vi "Image Processing.vi"(0 "File Path":path=path "C:/General AFM lithography program/Sample.ibw", 1 "Lithography Information":T2(array[cluster])=array7x3944[27608 elements], 2 "Crop?":bool, 3 "Crop Data":T3, 4 "Angle (degrees)":dbl, 5 "error in (no error)":errorcluster, 6 "Size":cluster{"Width":dbl, "Height":dbl}={"Width"=40.0, "Height"=40.0}, 7 "Page":i32=1, 11 "Resolution":i32=1024) -> (14 "Image Out":T4(plugin-control), 15 "Offset":T1={"X Offset (µm)"=-1.2812, "Y Offset (µm)"=5.2969}, 16 "Sample Size":cluster{"Width (µm)":dbl, "Height (µm)":dbl}={"Width (µm)"=40.0, "Height (µm)"=40.0}, 19 "error out":errorcluster)   [LabVIEW 2013]
uses:
  <vilib>/vision/NI_Vision_Development_Module.lvlib
panel:
  out "Suggested max":dbl
  out "Suggested min":dbl
  in  "Interested image data max":dbl(slide) min=-6.03287162448396e-08 max=6.376236569849425e-07 scale=-6.03287162448396e-08..6.376236569849425e-07
  in  "Interested image data min":dbl(slide) min=-6.03287162448396e-08 max=6.376236569849425e-07 scale=-6.03287162448396e-08..6.376236569849425e-07
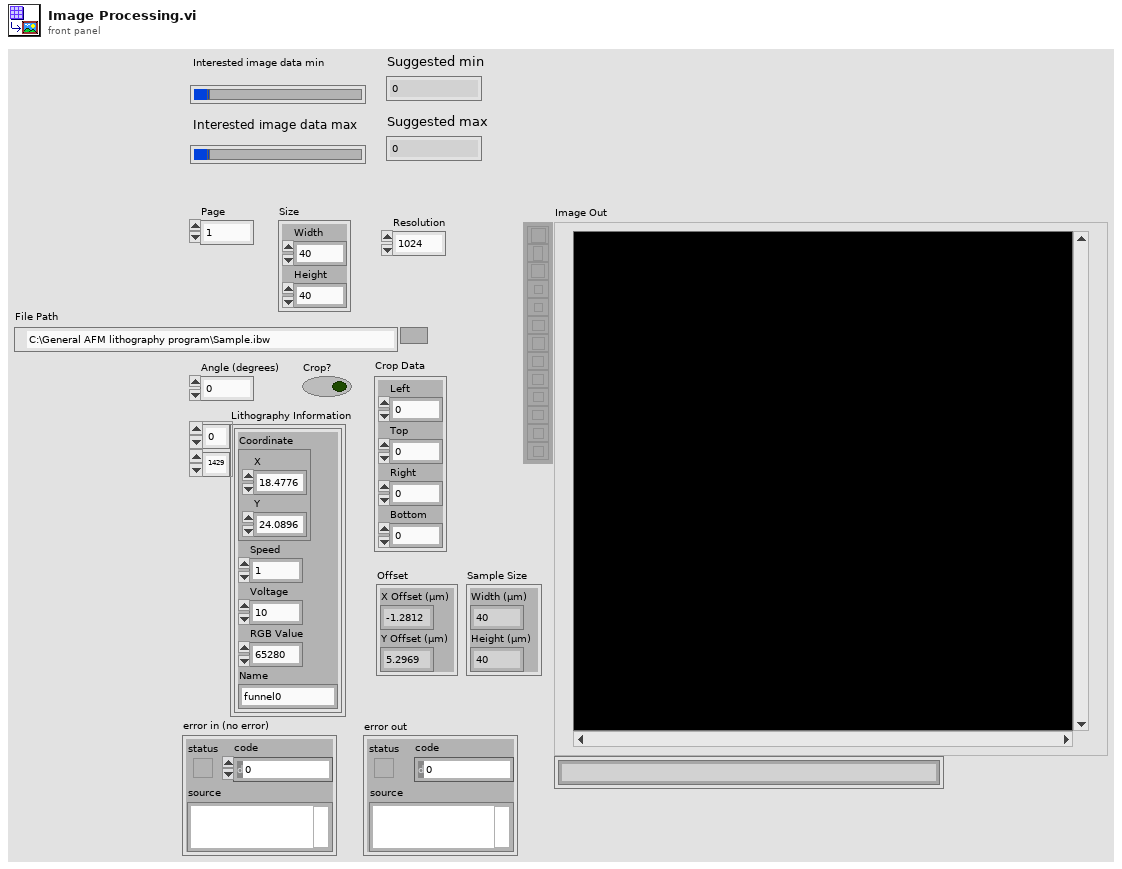
[diagram p1: front panel]
types:
  T1 = cluster{"X Offset (µm)":dbl, "Y Offset (µm)":dbl}
  T2 = cluster{"Coordinate":cluster{"X":dbl, "Y":dbl}, "Speed":dbl, "Voltage":dbl, "RGB Value":i32, "Name":string}[][]
  T3 = cluster{"Left":dbl, "Top":dbl, "Right":dbl, "Bottom":dbl}
  T4 = typedef "IMAQ Image.ctl" = refnum<image>
  T5 = typedef "Image Type" = u32
  T6 = cluster{"Coordinate":cluster{"X":dbl, "Y":dbl}, "Speed":dbl, "Voltage":dbl, "RGB Value":i32, "Name":string}
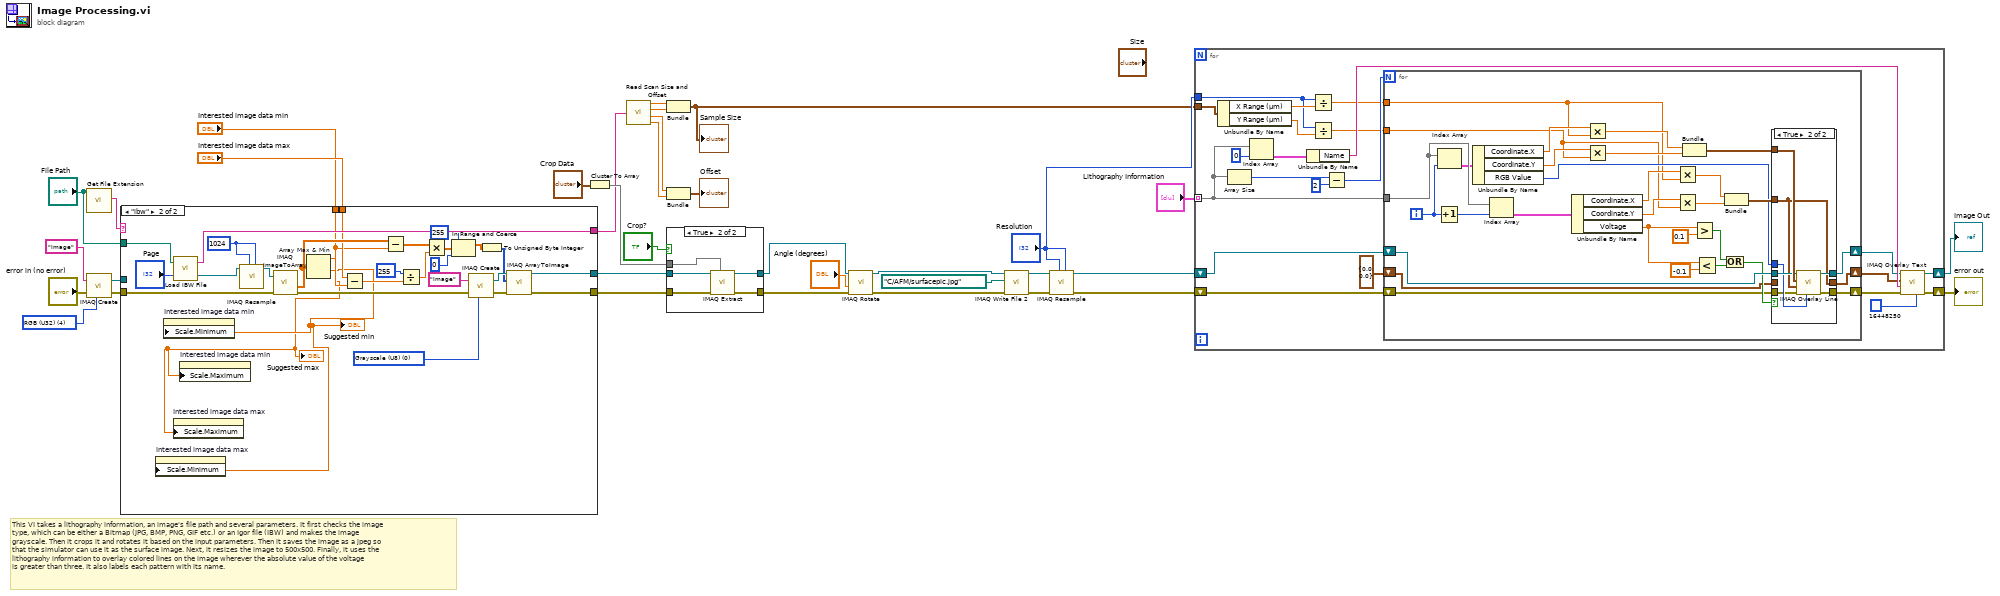
[diagram p0: block diagram]
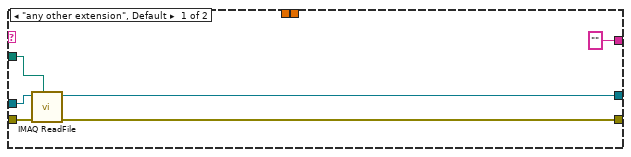
[diagram p2: hidden frame]
diagram:
  w34 = T5 4 items=["Grayscale (U8)", "Grayscale (I16)", "Grayscale (SGL)", "Complex (CSG)", "RGB (U32)", "HSL (U32)", "RGB (U64)", "Grayscale (U16)"] ("Image Type")
  # "This VI takes a lithography information, an image's file path and several parameters. It first checks the image \ntype, which can be either a Bitmap (JPG, BMP, PNG, GIF etc.) or an Igor file (IBW) and makes the image \ngrayscale. Then it crops it and rotates it based on the input parameters. Then it saves the image as a jpeg so \nthat the simulator can use it as the surface image. Next, it resizes the image to 500x500. Finally, it uses the \nlithography information to overlay colored lines on the image wherever the absolute value of the voltage \nis greater than three. It also labels each pattern with its name."
  n1 = call <vilib>:"Get File Extension.vi"("file"="File Path") -> ("lowercase file extension"=w21:string)  [unwired: 7 in, 3 out]
  n2 = call "IMAQ Create"("Image Name"="Image", "Image Type"=w34, "error in (no error)"="error in (no error)") -> ("New Image"=w33:T4, "error out"=w32:errorcluster)  [unwired: 2 in]
  n3 = case shown="\"ibw\"" w21 {
    tunnel: w33 -> [w41 _]
    tunnel: w32 -> [w40 w67]
    tunnel: [w39 w60] -> w31
    tunnel: [w38 w59] -> w30
    tunnel: "File Path" -> [w37 w69]
    tunnel: ["" ("Wave Note") w50] -> w10
    tunnel: "Interested image data max" -> [_ w49]
    tunnel: "Interested image data min" -> [_ w48]
    frame "any other extension", Default {
      n4 = call "IMAQ ReadFile"("File Path"=w37, "error in (no error)"=w40, "Image"=w41) -> ("error out"=w38:errorcluster, "Image Out"=w39:T4)  [unwired: 4 in, 3 out]
    }
    frame "ibw" {
      w57 = 1024 ("Y Resolution")
      w64 = T5 0 items=["Grayscale (U8)", "Grayscale (I16)", "Grayscale (SGL)", "Complex (CSG)", "RGB (U32)", "HSL (U32)", "RGB (U64)", "Grayscale (U16)"] ("Image Type")
      n5 = call "Load IBW File.vi"("Page"="Page", "file path (dialog if empty)"=w69) -> ("Image"=w56:T4, "Wave Note"=w50:string)
      n6 = call "IMAQ Resample"("X Resolution"=w57, "Y Resolution"=w57, "Image Src"=w56) -> ("Image Dst Out"=w55:T4)  [unwired: 7 in, 1 out]
      n7 = call "IMAQ ImageToArray"("error in (no error)"=w67, "Image"=w55) -> ("Image Pixels (Float)"=w66:sgl[][], "error out"=w61:errorcluster)  [unwired: 2 in, 3 out]
      n8 = Array Max & Min(array=w66) -> (max value=w42:sgl, min value=w43:sgl)  [unwired: 2 out]
      "Suggested min" <- w43
      "Suggested max" <- w42
      n9 = property on="Interested image data max" class="Slide (strict)"("Scale.Minimum"=w43) -> ()  [unwired: 2 in, 2 out]
      n10 = property on="Interested image data min" class="Slide (strict)"("Scale.Minimum"=w43) -> ()  [unwired: 2 in, 2 out]
      n11 = property on="Interested image data max" class="Slide (strict)"("Scale.Maximum"=w42) -> ()  [unwired: 2 in, 2 out]
      n12 = property on="Interested image data min" class="Slide (strict)"("Scale.Maximum"=w42) -> ()  [unwired: 2 in, 2 out]
      n13 = Subtract(x=w49, y=w48) -> (x-y=w53:dbl)
      n14 = Subtract(x=w66, y=w48) -> (x-y=w54:dbl[][])
      n15 = Divide(x=255, y=w53) -> (x/y=w51:dbl)
      n16 = Multiply(x=w54, y=w51) -> (x*y=w47:dbl[][])
      n17 = In Range and Coerce(upper limit=255, x=w47, lower limit=0) -> (coerced(x)=w44:dbl[][])  [unwired: 1 out]
      n18 = call "IMAQ Create"("Image Name"="Image", "Image Type"=w64, "error in (no error)"=w61) -> ("New Image"=w65:T4, "error out"=w62:errorcluster)  [unwired: 2 in]
      n19 = To Unsigned Byte Integer(number=w44) -> (unsigned 8bit integer=w63:u8[][])
      n20 = call "IMAQ ArrayToImage"("error in (no error)"=w62, "Image Pixels (U8)"=w63, "Image"=w65) -> ("error out"=w59:errorcluster, "Image Out"=w60:T4)  [unwired: 7 in]
    }
  }
  n21 = Cluster To Array(cluster="Crop Data") -> (array=w28:dbl[])
  n22 = call "Read Scan Size and Offset.vi"("Read in the string file"=w10) -> ("X Range (µm)"=w9:dbl, "Y Range (µm)"=w8:dbl, "X Offset (µm)"=w7:dbl, "Y Offset (µm)"=w6:dbl)  [unwired: 4 in]
  n23 = Bundle("X Range (µm)"=w9, "Y Range (µm)"=w8) -> (w3:cluster{"X Range (µm)":dbl, "Y Range (µm)":dbl})  [unwired: 1 in]
  "Sample Size" <- w3
  n24 = Bundle("X Offset (µm)"=w7, "Y Offset (µm)"=w6) -> (→"Offset":T1)  [unwired: 1 in]
  n25 = case shown="True" "Crop?" {
    tunnel: w31 -> [w71 w75]
    tunnel: w30 -> [w70 w74]
    tunnel: w28 -> [_ w76]
    tunnel: [w71 w72] -> w19
    tunnel: [w70 w73] -> w18
    frame False {
    }
    frame True {
      n26 = call "IMAQ Extract"("Optional Rectangle"=w76, "error in (no error)"=w74, "Image Src"=w75) -> ("error out"=w73:errorcluster, "Image Dst Out"=w72:T4)  [unwired: 7 in]
    }
  }
  n27 = call "IMAQ Rotate"("error in (no error)"=w18, "Angle (degrees)"="Angle (degrees)", "Image Src"=w19) -> ("error out"=w15:errorcluster, "Image Dst Out"=w16:T4)  [unwired: 7 in]
  n28 = call-poly "IMAQ Write File 2"("error in (no error)"=w15, "File Path"=path "C:/AFM/surfacepic.jpg", "Image"=w16) -> ("error out"=w13:errorcluster, "Image Out (duplicate)"=w14:T4)  [unwired: 7 in]
  n29 = call "IMAQ Resample"("X Resolution"="Resolution", "Y Resolution"="Resolution", "error in (no error)"=w13, "Image Src"=w14) -> ("error out"=w11:errorcluster, "Image Dst Out"=w12:T4)  [unwired: 6 in]
  n30 = for {
    tunnel: "Lithography Information" -> [w85] mode=indexing
    shift-right: [w87] -> w23
    shift-left: w12 -> [w93]
    shift-right: [w89] -> w26
    shift-left: w11 -> [w95]
    tunnel: "Resolution" -> [w78]
    tunnel: w3 -> [w77]
    n31 = Unbundle By Name(w77) -> ("X Range (µm)"=w80:dbl, "Y Range (µm)"=w79:dbl)
    n32 = Array Size(array=w85) -> (size(s)=w98:i32)
    n33 = Index Array(array=w85, index=0) -> (element=w83:T6)
    n34 = Unbundle By Name(w83) -> ("Name"=w92:string)
    n35 = Divide(x=w78, y=w80) -> (x/y=w82:dbl)
    n36 = Divide(x=w78, y=w79) -> (x/y=w81:dbl)
    n37 = Subtract(x=w98, y=2) -> (x-y=w96:i32)
    n38 = for {
      N: w96 -> [_]
      tunnel: w85 -> [w106]
      shift-right: [w114] -> w88
      shift-left: w93 -> [w123]
      shift-right: [w107] -> w90
      shift-left: w95 -> [w108]
      tunnel: w82 -> [w102]
      shift-right: [w101] -> w86
      shift-left: cluster{dbl, dbl} {0.0, 0.0} -> [w100]
      tunnel: w81 -> [w99]
      i -> [w105]
      n39 = Increment(x=w105) -> (x+1=w124:i32)
      n40 = Index Array(array=w106, index=w105) -> (element=w104:T6)
      n41 = Unbundle By Name(w104) -> ("Coordinate.X"=w128:dbl, "Coordinate.Y"=w127:dbl, "RGB Value"=w115:i32)
      n42 = Index Array(array=w106, index=w124) -> (element=w121:T6)
      n43 = Unbundle By Name(w121) -> ("Coordinate.X"=w119:dbl, "Coordinate.Y"=w120:dbl, "Voltage"=w103:dbl)
      n44 = Multiply(x=w128, y=w102) -> (x*y=w126:dbl)
      n45 = Multiply(x=w127, y=w99) -> (x*y=w125:dbl)
      n46 = Multiply(x=w119, y=w102) -> (x*y=w118:dbl)
      n47 = Multiply(x=w120, y=w99) -> (x*y=w117:dbl)
      n48 = Bundle(w126, w125) -> (w122:cluster{dbl, dbl})  [unwired: 1 in]
      n49 = Greater?(x=w103, y=0.1) -> (0:w111:bool)
      n50 = Less?(x=w103, y=-0.1) -> (x < y?=w110:bool)
      n51 = Or(x=w111, y=w110) -> (x .or. y?=w109:bool)
      n52 = Bundle(w118, w117) -> (w116:cluster{dbl, dbl})  [unwired: 1 in]
      n53 = case shown="True" w109 {
        tunnel: w123 -> [w131 w136]
        tunnel: w122 -> [_ w138]
        tunnel: w116 -> [_ w132]
        tunnel: w115 -> [_ w135]
        tunnel: [w131 w137] -> w114
        tunnel: w108 -> [w130 w134]
        tunnel: [w130 w133] -> w107
        tunnel: [w129 w132] -> w101
        tunnel: w100 -> [w129 _]
        frame False {
        }
        frame True {
          n54 = call "IMAQ Overlay Line"("Color"=w135, "error in (no error)"=w134, "End Point"=w132, "Start Point"=w138, "Image"=w136) -> ("error out"=w133:errorcluster, "Image Out"=w137:T4)  [unwired: 5 in]
        }
      }
    }
    n55 = call "IMAQ Overlay Text"("BG Color (Transparent)"=u32 16448250, "error in (no error)"=w90, "String"=w92, "Origin"=w86, "Image"=w88) -> ("error out"=w89:errorcluster, "Image Out"=w87:T4)  [unwired: 5 in]
  }
  "Image Out" <- w23
  "error out" <- w26
